vi "Configure Controlling E5091A.vi"(0 "VISA resource name":refnum<visa-resource-name>, 1 "Channel (1)":i32=1, 2 "Multiplexer (1)":i32=1, 3 "Control State (F: Disable)":bool, 5 "Property Display (F: Disable)":bool, 7 "Port 1 (0: A)":u16(ring) items=["A", "T1"], 9 "Port 2 (0: A)":u16(ring) items=["A", "T1"], 11 "error in (no error)":errorcluster, 12 "Port 3 (0: R1+)":u16(ring) items=["R1+", "R2+", "R3+"], 13 "Port 4 (0: R1-)":u16(ring) items=["R1-", "R2-", "R3-"], 14 "Control Lines (0)":i32) -> (4 "VISA resource name out":refnum<visa-resource-name>, 15 "error out":errorcluster)   [LabVIEW 2020, in "Agilent ENA Series.lvlib"]
doc: "Configures control of the Multiport Test Set (E5091A) accessory.\n\n<b>Note:</b>\nThis VI is not supported by the E5063A, E5080A and E5080B."
uses:
  <instrlib>/Agilent ENA Series/Agilent ENA Series.lvlib
panel:
  # "Note:\nThis VI is not supported by the \nE5063A, E5080A and E5080B."
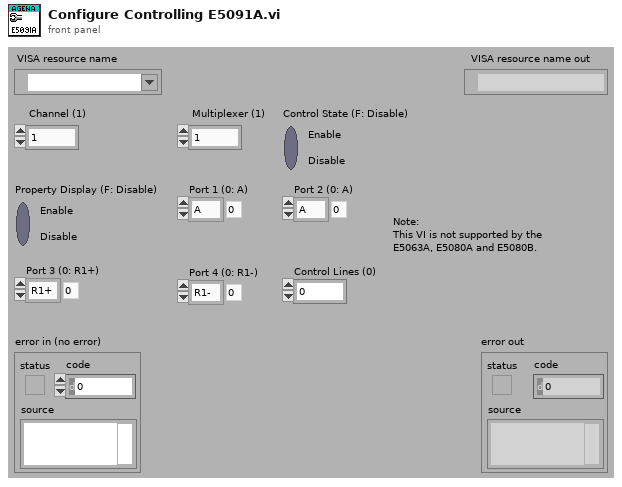
[diagram p1: front panel]
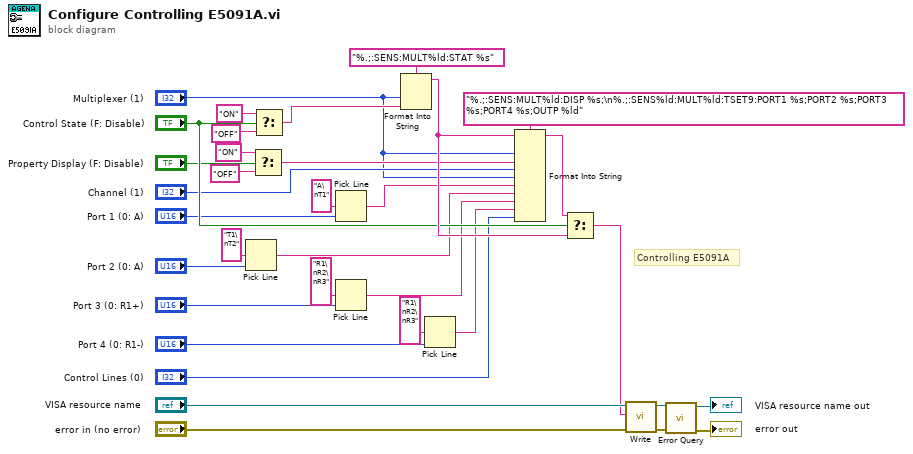
[diagram p0: block diagram]
diagram:
  # "Controlling E5091A"
  n1 = Pick Line(multi-line string="T1\nT2", line index="Port 2 (0: A)") -> (output string=w8:string)  [unwired: 1 in]
  n2 = Select(t="ON", s="Property Display (F: Disable)", f="OFF") -> (s? t:f=w20:string)
  n3 = Select(t="ON", s="Control State (F: Disable)", f="OFF") -> (s? t:f=w29:string)
  n4 = Pick Line(multi-line string="A\nT1", line index="Port 1 (0: A)") -> (output string=w15:string)  [unwired: 1 in]
  n5 = Pick Line(multi-line string="R1\nR2\nR3", line index="Port 3 (0: R1+)") -> (output string=w7:string)  [unwired: 1 in]
  n6 = Format Into String(format string="%.;:SENS:MULT%ld:STAT %s", "Multiplexer (1)", w29) -> (resulting string=w27:string)  [unwired: 2 in, 1 out]
  n7 = Pick Line(multi-line string="R1\nR2\nR3", line index="Port 4 (0: R1-)") -> (output string=w6:string)  [unwired: 1 in]
  n8 = Format Into String(format string="%.;:SENS:MULT%ld:DISP %s;\n%.;:SENS%ld:MULT%ld:TSET9:PORT1 %s;PORT2 %s;PORT3 %s;PORT4 %s;OUTP %ld", initial string=w27, "Multiplexer (1)", w20, "Channel (1)", "Multiplexer (1)", w15, w8, w7, w6, "Control Lines (0)") -> (resulting string=w25:string)  [unwired: 1 in, 1 out]
  n9 = Select(t=w25, s="Control State (F: Disable)", f=w27) -> (s? t:f=w26:string)
  n10 = call <instrlib>:"Write.vi"("error in (no error)"="error in (no error)", "String ()"=w26, "VISA resource name"="VISA resource name") -> ("error out"=w3:errorcluster, "VISA resource name out"=w4:refnum<visa-resource-name>)  [unwired: 6 in, 1 out]
  n11 = call <instrlib>:"Error Query.vi"("error in (no error)"=w3, "VISA resource name"=w4) -> ("error out"=→"error out":errorcluster, "VISA resource name out"=→"VISA resource name out":refnum<visa-resource-name>)  [unwired: 6 in, 2 out]
